vi "new alias tree.vi"(5 "allow multi-select":bool, 7 "show checkbox":bool, 8 "error in (no error)":errorcluster, 10 "sdf path":string, 11 "tree ref":refnum<k24>) -> (0 "error out":errorcluster, 3 "alias-tree":refnum<class "alias-tree.lvclass">)   [LabVIEW 2017, in "vs-tree-utility.lvlib" / "alias-tree.lvclass"]
uses:
  alias-tree.lvclass
  NationalInstruments.VeriStand.SystemStorageUI
  alias-tree.lvclass/alias-tree.ctl
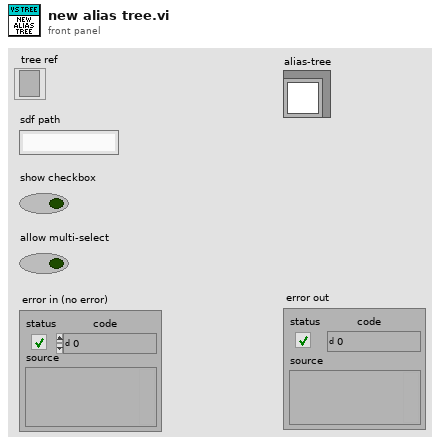
[diagram p1: front panel]
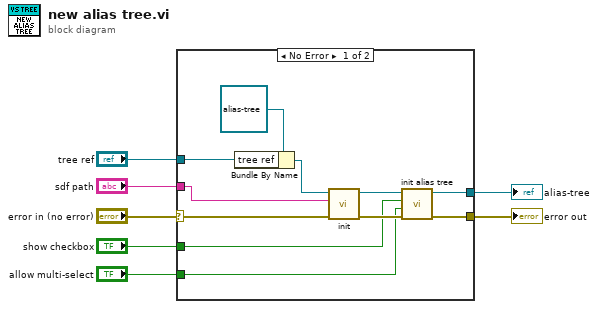
[diagram p0: block diagram]
diagram:
  n1 = case shown="No Error" "error in (no error)" {
    selector: "error in (no error)" -> [w18 w19]
    tunnel: [w10 w19] -> w6
    tunnel: "tree ref" -> [w16 _]
    tunnel: "sdf path" -> [w15 _]
    tunnel: [w11 _] -> w3
    tunnel: "allow multi-select" -> [w9 _]
    tunnel: "show checkbox" -> [w8 _]
    frame No Error {
      n2 = Bundle By Name(cluster=refnum<class "alias-tree.lvclass"> refnum ("vs-tree-utility.lvlib:alias-tree.lvclass"), "tree ref"=w16) -> (w14:refnum<class "alias-tree.lvclass">)
      n3 = call-dynamic "init.vi"("error in (no error)"=w18, "sdf path"=w15, "abstract-tree in"=w14) -> ("error out"=w13:errorcluster, "abstract-tree out"=w12:refnum<class "alias-tree.lvclass">)  [unwired: 7 in]
      n4 = call-dynamic "init alias tree.vi"("error in (no error)"=w13, "allow multi-select"=w9, "show checkbox"=w8, "alias-tree in"=w12) -> ("error out"=w10:errorcluster, "alias-tree out"=w11:refnum<class "alias-tree.lvclass">)  [unwired: 6 in]
    }
    frame Error {
    }
  }
  "error out" <- w6
  "alias-tree" <- w3
